vi "Create UA Server.vi"(8 "error in (no error)":errorcluster, 9 "LDS Server URL in (opt)":string, 11 "OPCUA Setting In":T2) -> (0 "error out":errorcluster, 2 "Server endpoint  URL out":string, 3 "OPC UA server refnum out":T1)   [LabVIEW 2024]
uses:
  OPCUA/OPCUA Setting.ctl
  <vilib>/OPCUA/controls/OPC UA Server Refnum.ctl
  <vilib>/OPCUA/controls/Supported Security Policies.ctl
  <vilib>/OPCUA/NI OPC UA Server.lvlib
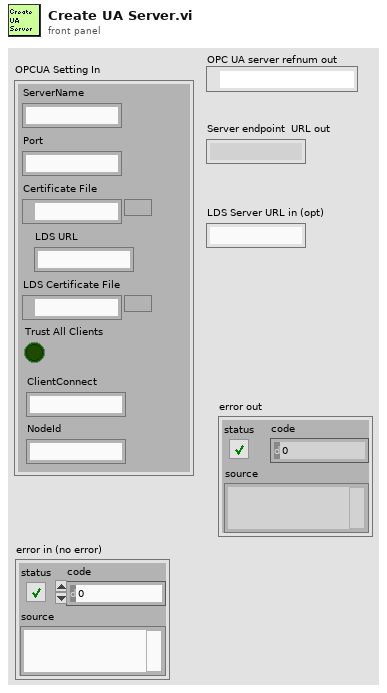
[diagram p1: front panel]
types:
  T1 = typedef "OPC UA Server Refnum.ctl" = refnum<k21>
  T2 = typedef "OPCUA Setting.ctl" = cluster{"ServerName":string, "Port":string, "Certificate File":path, "LDS URL":string, "LDS Certificate File":path, "Trust All Clients":bool, "ClientConnect":string, "NodeId":string}
  T3 = typedef "Supported Security Policies.ctl" = cluster{"None":bool, "Sign with Basic128Rsa15":bool, "Sign and Encrypt with Basic128Rsa15":bool, "Sign with Basic256":bool, "Sign and Encrypt with Basic256":bool}
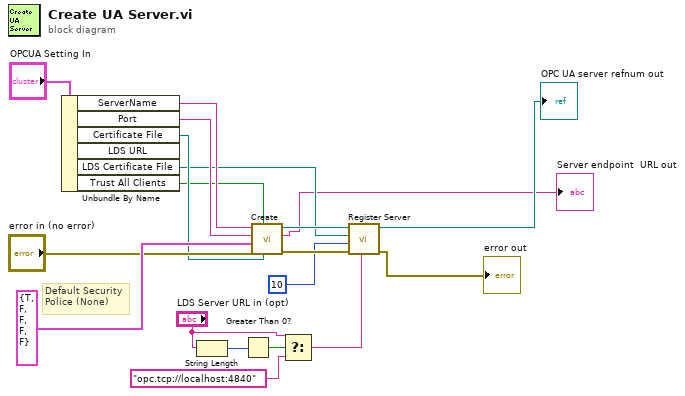
[diagram p0: block diagram]
diagram:
  # "Default Security\nPolice (None)"
  n1 = Unbundle By Name("OPCUA Setting In") -> ("ServerName"=w18:string, "Port"=w17:string, "Certificate File"=w14:path, "LDS Certificate File"=w10:path, "Trust All Clients"=w13:bool)  [unwired: 1 out]
  n2 = String Length(string="LDS Server URL in (opt)") -> (length=w8:i32)
  n3 = Greater Than 0?(x=w8) -> (x > 0?=w7:bool)
  n4 = call <vilib>:"Create.vi"("server certificate file"=w14, "trust all clients (F)"=w13, "error in (no error)"="error in (no error)", "supported security policies (None)"=T3 {"None"=TRUE, "Sign with Basic128Rsa15"=FALSE, "Sign and Encrypt with Basic128Rsa15"=FALSE, "Sign with Basic256"=FALSE, "Sign and Encrypt with Basic256"=FALSE}, "TCP port (49580)"=w17, "OPC UA server name"=w18) -> ("error out"=w11:errorcluster, "server endpoint URL"=→"Server endpoint  URL out":string, "OPC UA server refnum out"=w12:T1)  [unwired: 3 in]
  n5 = Select(t="LDS Server URL in (opt)", s=w7, f="opc.tcp://localhost:4840" ("local discovery server URL (opc.tcp://localhost:4840)")) -> (s? t:f=w4:string)
  n6 = call <vilib>:"Register Server.vi"("local discovery server URL (opc.tcp://localhost:4840)"=w4, "error in (no error)"=w11, "register rate (10 min)"=u32 10, "local discovery server certificate file"=w10, "OPC UA server refnum in"=w12) -> ("error out"=→"error out":errorcluster, "OPC UA server refnum out"=→"OPC UA server refnum out":T1)  [unwired: 5 in]
